vi "Finish Update.vi"(8 "instVIref":T1, 11 "target in":refnum<class "NetCPU.lvclass">) -> (3 "target out":refnum<class "NetCPU.lvclass">)   [LabVIEW 2020, in "NI_TargetHelper.lvlib" / "NetCPU.lvclass"]
uses:
  <vilib>/TargetSupport/NI_TargetHelper/NetCPU/NetCPU.lvclass
  <vilib>/TargetSupport/NI_TargetHelper/Instance VIref.ctl
  <vilib>/TargetSupport/NI_TargetHelper/NetCPU/NetCPU.lvclass/NetCPU.ctl
  08a85ab3-64aa-304c-91f7-0345f7456145.vi
  <vilib>/UserTags/Get User VI Tag.vi
  <vilib>/TargetSupport/NI_TargetHelper/NI_TargetHelper.lvlib
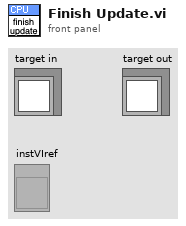
[diagram p1: front panel]
types:
  T1 = typedef "NI_TargetHelper.lvlib/Instance VIref.ctl" = refnum<vi>
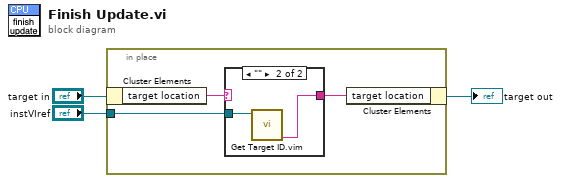
[diagram p0: block diagram]
diagram:
  n1 = in-place {
    in-place-border: "instVIref" -> [w4]
    n2 = in-place-cluster #1("target in") -> ("target location"=w6:string)
    n3 = case shown="\"\"" w6 {
      selector: w6 -> [w7 _]
      tunnel: [w7 w8] -> w5
      tunnel: w4 -> [_ w9]
      frame Default {
      }
      frame "" {
        n4 = call "Get Target ID.vim"("ref in"=w9) -> ("target ID"=w8:string)  [unwired: 9 in, 1 out]
      }
    }
    n5 = in-place-cluster #1("target location"=w5) -> (→"target out":refnum<class "NetCPU.lvclass">)
  }
